vi "ief_open_connections.vi"(3 "error in (no error)":errorcluster, 4 "NumberOfAxes":u16, 5 "Tagprefix in":refnum<k21>) -> (0 "error out (no error)":errorcluster, 2 "Tagprefix out":refnum<k21>)   [LabVIEW 2015, in "IEF Werner.lvlib"]
doc: "Opens the SV connection to all necessary variables."
uses:
  IEF Werner.lvlib
  Packages/CSPP_Core/Libraries/Base/FGV Action.ctl
  Packages/CSPP_Core/Libraries/Base/CS++Base.lvlib
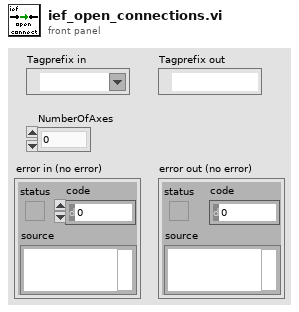
[diagram p1: front panel]
types:
  T1 = typedef "CS++Base.lvlib/FGV Action.ctl" = enum16{"add", "replace", "read", "remove", "reset", "get attributes"}
  T2 = cluster{"Read Access":enum8{"Allowed", "Required", "None"}, "Write Access":enum8{"Allowed", "Required", "None"}}
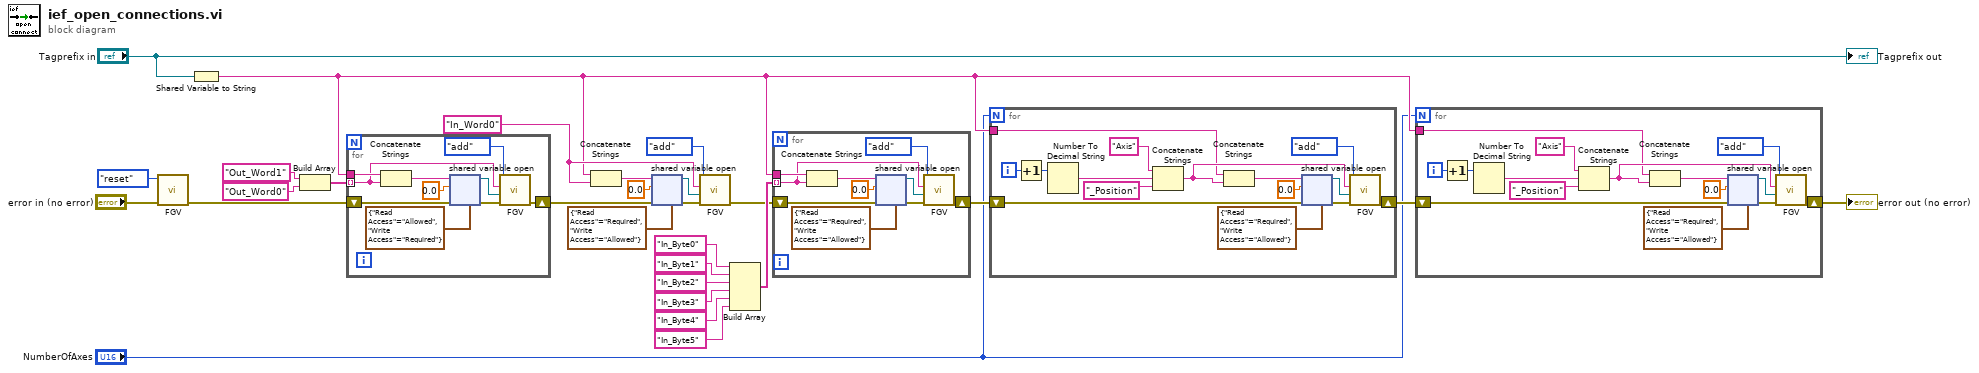
[diagram p0: block diagram]
diagram:
  w6 = "In_Word0" ("string")
  n1 = call "FGV.vi"("Error In"="error in (no error)", "Action (read)"=FGV_Action."reset") -> ("Error Out"=w11:errorcluster)  [unwired: 5 in, 4 out]
  n2 = Shared Variable to String(1:"Tagprefix in") -> (0:w2:string)
  n3 = Build Array("Out_Word1", "Out_Word0") -> (w25:string[])
  n4 = for {
    shift-right: [w32] -> w14
    shift-left: w11 -> [w38]
    tunnel: w25 -> [w29] mode=indexing
    tunnel: w2 -> [w36]
    n5 = Concatenate Strings(w36, w29) -> (w35:string)
    n6 = shared-variable-open(w35, w38, 0.0, T2 {"Read Access"=enum."Allowed", "Write Access"=enum."Required"} ("access")) -> (w31:refnum<k21>, w33:errorcluster)
    n7 = call "FGV.vi"("Error In"=w33, "Data in"=w31, "Attribute Name"=w29, "Action (read)"=FGV_Action."add") -> ("Error Out"=w32:errorcluster)  [unwired: 3 in, 4 out]
  }
  n8 = Concatenate Strings(w2, w6) -> (w16:string)
  n9 = shared-variable-open(w16, w14, 0.0, T2 {"Read Access"=enum."Required", "Write Access"=enum."Allowed"} ("access")) -> (w8:refnum<k21>, w10:errorcluster)
  n10 = call "FGV.vi"("Error In"=w10, "Data in"=w8, "Attribute Name"=w6, "Action (read)"=FGV_Action."add") -> ("Error Out"=w9:errorcluster)  [unwired: 3 in, 4 out]
  n11 = Build Array("In_Byte0" ("string"), "In_Byte1" ("string"), "In_Byte2" ("string"), "In_Byte3" ("string"), "In_Byte4", "In_Byte5") -> (w18:string[])
  n12 = for {
    shift-right: [w42] -> w5
    shift-left: w9 -> [w48]
    tunnel: w18 -> [w39] mode=indexing
    tunnel: w2 -> [w46]
    n13 = Concatenate Strings(w46, w39) -> (w45:string)
    n14 = shared-variable-open(w45, w48, 0.0, T2 {"Read Access"=enum."Required", "Write Access"=enum."Allowed"} ("access")) -> (w41:refnum<k21>, w43:errorcluster)
    n15 = call "FGV.vi"("Error In"=w43, "Data in"=w41, "Attribute Name"=w39, "Action (read)"=FGV_Action."add") -> ("Error Out"=w42:errorcluster)  [unwired: 3 in, 4 out]
  }
  n16 = for {
    N: "NumberOfAxes" -> [_]
    shift-right: [w59] -> w3
    shift-left: w5 -> [w63]
    tunnel: w2 -> [w49]
    i -> [w55]
    n17 = Increment(x=w55) -> (x+1=w54:i32)
    n18 = Number To Decimal String(number=w54) -> (decimal integer string=w56:string)  [unwired: 1 in]
    n19 = Concatenate Strings("Axis" ("string"), w56, "_Position" ("string")) -> (w51:string)
    n20 = Concatenate Strings(w49, w51) -> (w50:string)
    n21 = shared-variable-open(w50, w63, 0.0, T2 {"Read Access"=enum."Required", "Write Access"=enum."Allowed"} ("access")) -> (w58:refnum<k21>, w60:errorcluster)
    n22 = call "FGV.vi"("Error In"=w60, "Data in"=w58, "Attribute Name"=w51, "Action (read)"=FGV_Action."add") -> ("Error Out"=w59:errorcluster)  [unwired: 3 in, 4 out]
  }
  n23 = for {
    N: "NumberOfAxes" -> [_]
    shift-right: [w74] -> w4
    shift-left: w3 -> [w78]
    tunnel: w2 -> [w64]
    i -> [w70]
    n24 = Increment(x=w70) -> (x+1=w69:i32)
    n25 = Number To Decimal String(number=w69) -> (decimal integer string=w71:string)  [unwired: 1 in]
    n26 = Concatenate Strings("Axis" ("string"), w71, "_Position" ("string")) -> (w66:string)
    n27 = Concatenate Strings(w64, w66) -> (w65:string)
    n28 = shared-variable-open(w65, w78, 0.0, T2 {"Read Access"=enum."Required", "Write Access"=enum."Allowed"} ("access")) -> (w73:refnum<k21>, w75:errorcluster)
    n29 = call "FGV.vi"("Error In"=w75, "Data in"=w73, "Attribute Name"=w66, "Action (read)"=FGV_Action."add") -> ("Error Out"=w74:errorcluster)  [unwired: 3 in, 4 out]
  }
  "error out (no error)" <- w4
  "Tagprefix out" <- "Tagprefix in"
